vi "Read Verbose.vi"(8 "error in (no error)":errorcluster, 11 "Test Report in":refnum<class "Test Report.lvclass">) -> (0 "error out":errorcluster, 2 "Verbose":bool, 3 "Test Report out":refnum<class "Test Report.lvclass">)   [LabVIEW 2020, in "Caraya.lvlib" / "Test Report.lvclass"]
uses:
  Test Report.lvclass
  Test Report.lvclass/Test Report.ctl
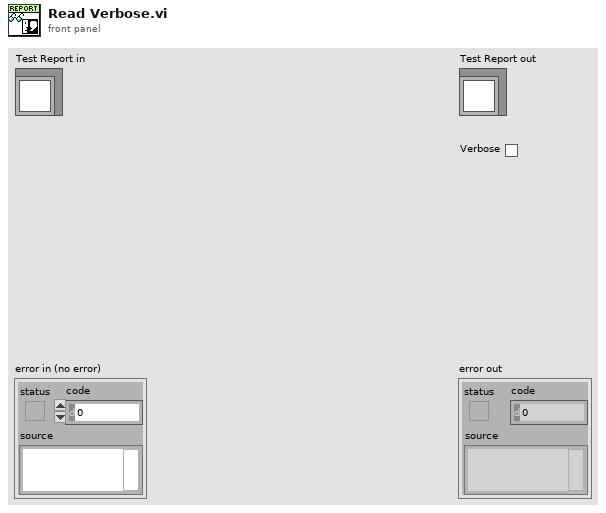
[diagram p1: front panel]
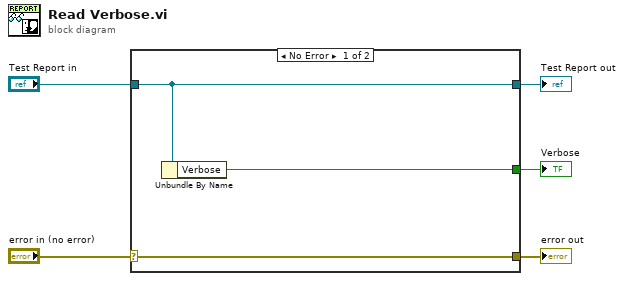
[diagram p0: block diagram]
diagram:
  n1 = case shown="No Error" "error in (no error)" {
    selector: "error in (no error)" -> [w8 w9]
    tunnel: [w8 w9] -> w4
    tunnel: [w7 w10] -> w2
    tunnel: "Test Report in" -> [w7 w10]
    tunnel: [w6 _] -> w1
    frame No Error {
      n2 = Unbundle By Name(w7) -> ("Verbose"=w6:bool)
    }
    frame Error {
    }
  }
  "error out" <- w4
  "Test Report out" <- w2
  "Verbose" <- w1
